vi "Config_AI_Module_NI_0_10V.vi"(8 "error in (no error)":errorcluster, 10 "MODULE NAME":string, 11 "Refnum in":refnum<k21>) -> (0 "error out":errorcluster, 3 "Refnum out":refnum<k21>)   [LabVIEW 2019]
uses:
  <vilib>/DAQmx/create/channels.llb/DAQmx Create Channel (AI-Voltage-Basic).vi
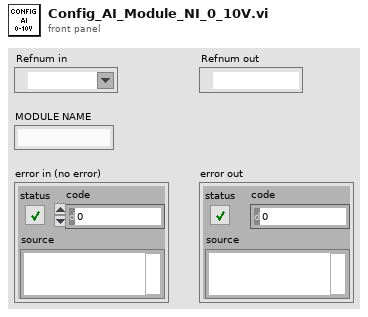
[diagram p1: front panel]
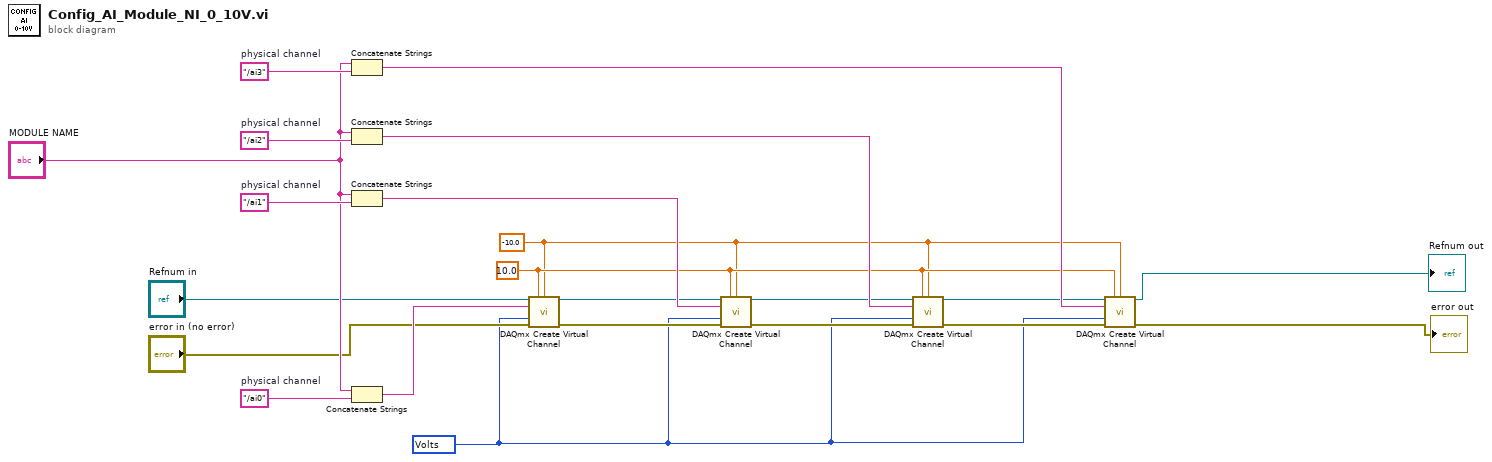
[diagram p0: block diagram]
diagram:
  w5 = 10348 items=["Volts"=10348, "From Custom Scale"=10065] ("units")
  w3 = -10.0 ("minimum value")
  w4 = 10.0 ("maximum value")
  w21 = "/ai3"  # physical channel
  w19 = "/ai2"  # physical channel
  w17 = "/ai1"  # physical channel
  w14 = "/ai0"  # physical channel
  n1 = Concatenate Strings("MODULE NAME", w21) -> (w22:string)
  n2 = Concatenate Strings("MODULE NAME", w19) -> (w20:string)
  n3 = Concatenate Strings("MODULE NAME", w17) -> (w18:string)
  n4 = Concatenate Strings("MODULE NAME", w14) -> (w15:string)
  n5 = call-poly <vilib>:"DAQmx Create Virtual Channel.vi"("task in"="Refnum in", "maximum value"=w4, "minimum value"=w3, "physical channels"=w15, "units"=w5, "error in"="error in (no error)") -> ("task out"=w9:refnum<k21>, "error out"=w8:errorcluster)  [unwired: 8 in]
  n6 = call-poly <vilib>:"DAQmx Create Virtual Channel.vi"("task in"=w9, "maximum value"=w4, "minimum value"=w3, "physical channels"=w18, "units"=w5, "error in"=w8) -> ("task out"=w11:refnum<k21>, "error out"=w10:errorcluster)  [unwired: 8 in]
  n7 = call-poly <vilib>:"DAQmx Create Virtual Channel.vi"("task in"=w11, "maximum value"=w4, "minimum value"=w3, "physical channels"=w20, "units"=w5, "error in"=w10) -> ("task out"=w13:refnum<k21>, "error out"=w12:errorcluster)  [unwired: 8 in]
  n8 = call-poly <vilib>:"DAQmx Create Virtual Channel.vi"("task in"=w13, "maximum value"=w4, "minimum value"=w3, "physical channels"=w22, "units"=w5, "error in"=w12) -> ("task out"=→"Refnum out":refnum<k21>, "error out"=→"error out":errorcluster)  [unwired: 8 in]
